vi "Set Array of LogicOut.vi"(8 "error in (no error)":errorcluster, 10 "Array of LogicOut":T1[](array[typedef]), 11 "VacuumLines Configuration in":refnum<class "VacuumLines Configuration.lvclass">) -> (0 "error out":errorcluster, 3 "VacuumLines Configuration out":refnum<class "VacuumLines Configuration.lvclass">)   [LabVIEW 2016, in "Hardware.lvlib" / "VacuumLine.lvlib" / "VacuumLines Configuration.lvclass"]
uses:
  <userlib>/Common Components/Hardware/Abstract System/VacuumLine/VacuumLines Configuration/VacuumLines Configuration.lvclass
  <userlib>/Common Components/Hardware/Abstract System/VacuumLine/VacuumLines/LogicOut.ctl
  <userlib>/Common Components/Hardware/Abstract System/VacuumLine/VacuumLines Configuration/VacuumLines Configuration.lvclass/VacuumLines Configuration.ctl
  <userlib>/Common Components/Hardware/Abstract System/VacuumLine/VacuumLines/VacuumLines.lvclass/VacuumLines.ctl
  <userlib>/Common Components/Hardware/Abstract System/VacuumLine/VacuumLines/VacuumLines.lvclass
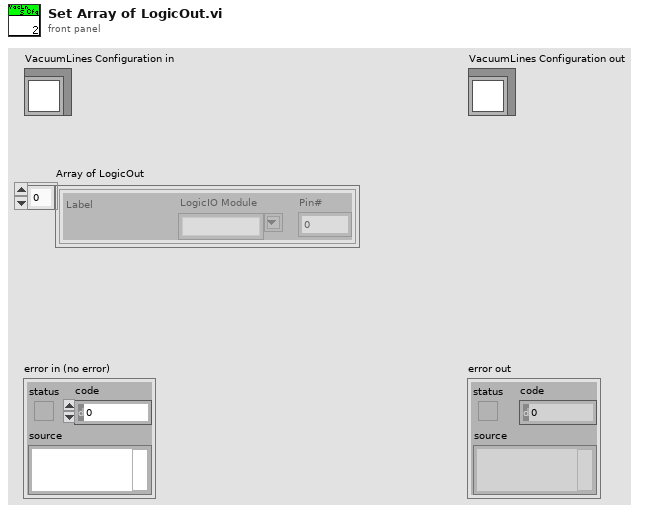
[diagram p1: front panel]
types:
  T1 = typedef "Hardware.lvlib/VacuumLine.lvlib/VacuumLines.lvclass/LogicOut.ctl" = cluster{"Label":string, "LogicIO Module":string, "Pin#":u8}
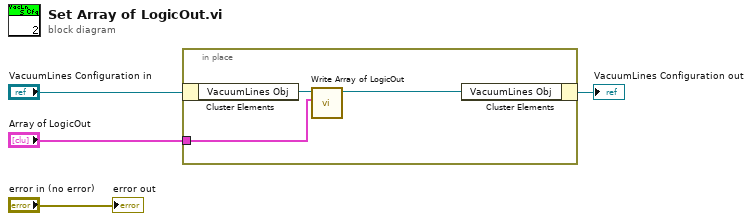
[diagram p0: block diagram]
diagram:
  n1 = in-place {
    in-place-border: "Array of LogicOut" -> [w5]
    n2 = in-place-cluster #1("VacuumLines Configuration in") -> ("VacuumLines Obj"=w7:refnum<class "VacuumLines.lvclass">)
    n3 = call <userlib>:"Write Array of LogicOut.vi"("Array of LogicOut"=w5, "VacuumLines in"=w7) -> ("VacuumLines out"=w6:refnum<class "VacuumLines.lvclass">)  [unwired: 9 in]
    n4 = in-place-cluster #1("VacuumLines Obj"=w6) -> (→"VacuumLines Configuration out":refnum<class "VacuumLines Configuration.lvclass">)
  }
  "error out" <- "error in (no error)"
